vi "GcolorVar.vi"() -> ()   [LabVIEW 2010]
panel:
  in  "Bit Shift":u16
  in  "Type of Bayer":u32
  in  "Blue Offset":dbl format="%.2f"
  in  "Green Offset":dbl format="%.2f"
  in  "Red Offset":dbl format="%.2f"
  in  "Blue Gain":dbl format="%.2f"
  in  "Green Gain":dbl format="%.2f"
  in  "Red Gain":dbl format="%.2f"
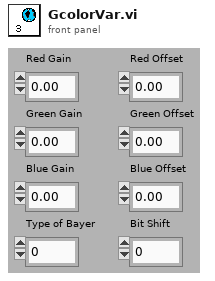
[diagram p1: front panel]
diagram:
